vi "Configure Communication.vi"() -> (0 "error out":errorcluster, 3 "Communication Channel.lvclass":refnum<class "Communication Channel.lvclass">)   [LabVIEW 2014, in "Communication Channel.lvclass"]
uses:
  Communication Channel.lvclass
  <vilib>/Skyline/Tag/Shared/typedefs/DataType.ctl
  Communication Channel.lvclass/Communication Channel.ctl
  <vilib>/Skyline/Configuration/Configuration HTTP_class/Open Configuration HTTP.vi
  <vilib>/Skyline/Tag/Wrapper/Wrapper HTTP_class/Open Tag HTTP.vi
  <vilib>/Skyline/Tag/Wrapper/Wrapper_class/NI Skyline Tag.lvclass
  <vilib>/Skyline/Tag/Wrapper/Wrapper HTTP_class/NI Skyline Tag HTTP.lvclass
  <vilib>/Skyline/Configuration/Configuration_class/NI Skyline Configuration.lvclass
  <vilib>/Skyline/Configuration/Configuration HTTP_class/NI Skyline Configuration HTTP.lvclass
  <vilib>/Skyline/Tag/Shared/NI Skyline Tag.lvlib
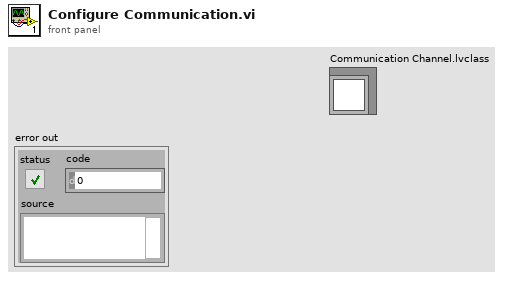
[diagram p1: front panel]
types:
  T1 = typedef "NI Skyline Tag.lvlib/DataType.ctl" = enum32{"Double", "I32", "String", "Boolean", "U64", "Timestamp"}
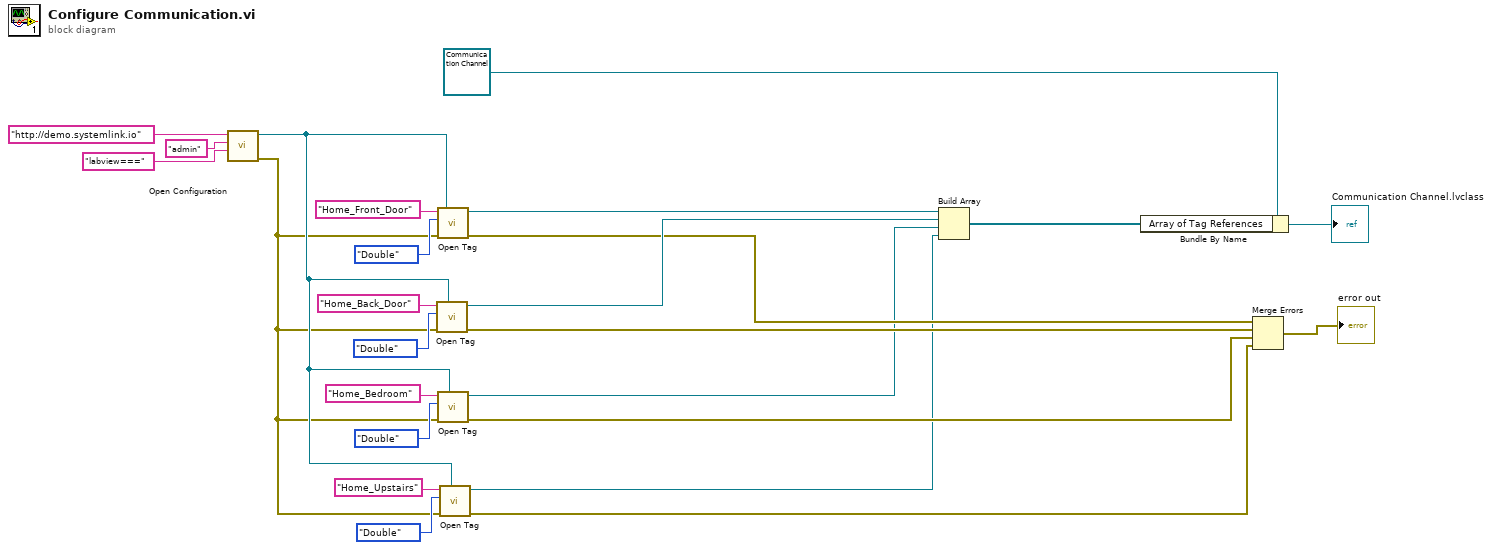
[diagram p0: block diagram]
diagram:
  n1 = call-poly <vilib>:"Open Configuration.vi"("password"="labview===" ("server url"), "username"="admin" ("server url"), "server url"="http://demo.systemlink.io") -> ("error out"=w3:errorcluster, "HTTP configuration out"=w4:refnum<class "NI Skyline Configuration HTTP.lvclass">)  [unwired: 7 in]
  n2 = call-poly <vilib>:"Open Tag.vi"("configuration"=w4, "error in (no error)"=w3, "Data Type"=DataType."Double", "path"="Home_Back_Door") -> ("error out"=w12:errorcluster, "tag out"=w14:refnum<class "NI Skyline Tag.lvclass">)  [unwired: 6 in]
  n3 = call-poly <vilib>:"Open Tag.vi"("configuration"=w4, "error in (no error)"=w3, "Data Type"=DataType."Double", "path"="Home_Front_Door") -> ("error out"=w13:errorcluster, "tag out"=w19:refnum<class "NI Skyline Tag.lvclass">)  [unwired: 6 in]
  n4 = call-poly <vilib>:"Open Tag.vi"("configuration"=w4, "error in (no error)"=w3, "Data Type"=DataType."Double", "path"="Home_Bedroom") -> ("error out"=w7:errorcluster, "tag out"=w8:refnum<class "NI Skyline Tag.lvclass">)  [unwired: 6 in]
  n5 = call-poly <vilib>:"Open Tag.vi"("configuration"=w4, "error in (no error)"=w3, "Data Type"=DataType."Double", "path"="Home_Upstairs") -> ("error out"=w2:errorcluster, "tag out"=w1:refnum<class "NI Skyline Tag.lvclass">)  [unwired: 6 in]
  n6 = Build Array(w19, w14, w8, w1) -> (w18:refnum<class "NI Skyline Tag.lvclass">[])
  n7 = Bundle By Name(cluster=refnum<class "Communication Channel.lvclass"> refnum ("Communication Channel.lvclass"), "Array of Tag References"=w18) -> (→"Communication Channel.lvclass":refnum<class "Communication Channel.lvclass">)
  n8 = Merge Errors(w13, w12, w7, w2) -> (→"error out":errorcluster)
